vi "AtDome_getEvent_detailedState.vi"(8 "error in (no error)":errorcluster, 11 "logevent_detailedState_Ctl":T1) -> (0 "error out":errorcluster, 2 "function return":i32, 3 "logevent_detailedState_Ctl out":T1)   [LabVIEW 2016, in "SALLV_AtDome.lvlib"]
doc: "int AtDome_shm_getEvent_detailedStateLV(AtDome_logevent_detailedStateLV *logevent_detailedState_Ctl );"
uses:
  SALLV_AtDome.lvlib
  DataTypes/logevent_detailedState.ctl
  SALLV_AtDome.so
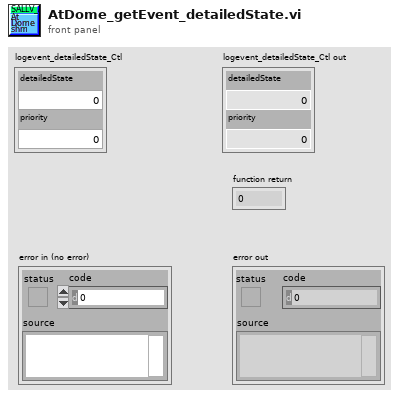
[diagram p1: front panel]
types:
  T1 = typedef "SALLV_AtDome.lvlib/logevent_detailedState.ctl" = cluster{"detailedState":i32, "priority":i32}
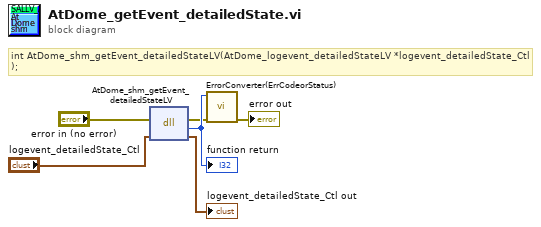
[diagram p0: block diagram]
diagram:
  # "int AtDome_shm_getEvent_detailedStateLV(AtDome_logevent_detailedStateLV *logevent_detailedState_Ctl );"
  n1 = dll-call lib="home/andres/Desktop/SAL_AtDome/SALLV_AtDome.*" fn="AtDome_shm_getEvent_detailedStateLV"(error in="error in (no error)", "logevent_detailedState_Ctl"="logevent_detailedState_Ctl") -> (error out=w2:errorcluster, w6:i32, "logevent_detailedState_Ctl"=→"logevent_detailedState_Ctl out":T1)  [unwired: 2 in, 1 out]
  "function return" <- w6
  n2 = call "ErrorConverter(ErrCodeorStatus).vi"("error in (no error)"=w2, "error code"=w6) -> ("error out"=→"error out":errorcluster)  [unwired: 9 in]
